vi "onTestExecution.vi"(7 "Name":string, 8 "error in (no error)":errorcluster, 11 "Test Runner.AllAsserts in":refnum<class "Test Runner.AllAsserts.lvclass">) -> (0 "error out":errorcluster, 3 "Test Runner.AllAsserts out":refnum<class "Test Runner.AllAsserts.lvclass">)   [LabVIEW 2013, in "Test Runner.AllAsserts.lvclass"]
uses:
  Test Runner.AllAsserts.lvclass
  classes/Test/Test.lvclass
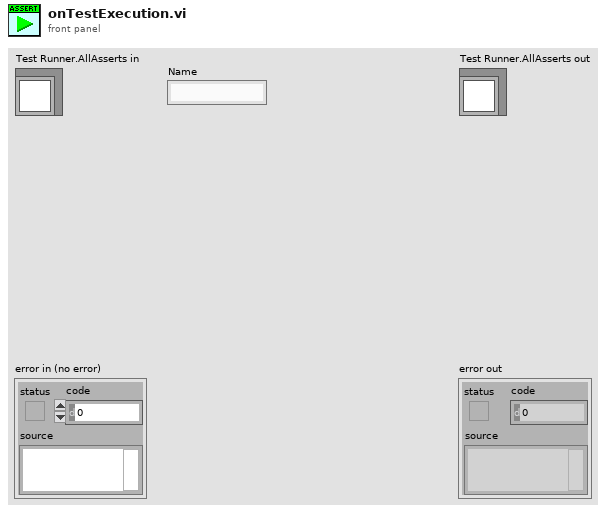
[diagram p1: front panel]
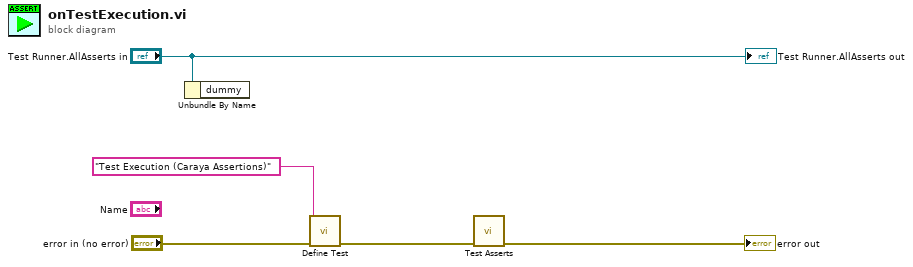
[diagram p0: block diagram]
diagram:
  n1 = Unbundle By Name("Test Runner.AllAsserts in") -> ()  [unwired: 1 out]
  n2 = call "Define Test.vi"("error in (no error)"="error in (no error)", "Label (VI Title)"="Test Execution (Caraya Assertions)") -> ("error out"=w2:errorcluster)  [unwired: 9 in]
  n3 = call "Test Asserts.vi"("error in (no error)"=w2) -> ("error out"=→"error out":errorcluster)  [unwired: 10 in]
  "Test Runner.AllAsserts out" <- "Test Runner.AllAsserts in"
